vi "vol_path_by_id.get.vi"(8 "error in (no error)":errorcluster, 10 "vol id":i32, 11 "manager_daemon":refnum<class "manager_daemon.lvclass">) -> (0 "error out":errorcluster, 2 "Path":path, 3 "manager_daemon out":refnum<class "manager_daemon.lvclass">)   [LabVIEW 2024, in "manager_daemon.lvclass"]
uses:
  manager_daemon.lvclass
  manager_daemon.lvclass/manager_daemon.ctl
  type_defs/cmd--enum.ctl
  type_defs/msg--cluster.ctl
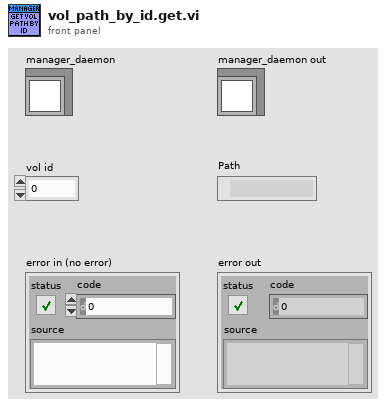
[diagram p1: front panel]
types:
  T1 = typedef "manager_daemon.lvclass/cmd--enum.ctl" = enum16{"init", "run", "load binaries", "build binaries", "save binaries", "return vol path by id", "display info", "apply filter", "add volume", "add issues", "add issue", "delete volume", "delete issues", "exit"}
  T2 = typedef "manager_daemon.lvclass/msg--cluster.ctl" = cluster{"cmd":T1, "data":variant}
  T3 = cluster{"vol id":i32, "notifier out":refnum<notifier>}
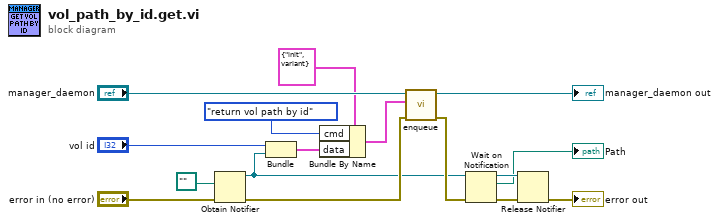
[diagram p0: block diagram]
diagram:
  n1 = Obtain Notifier(notification data type=path "", error in (no error)="error in (no error)") -> (notifier out=w5:refnum<notifier>, error out=w7:errorcluster)  [unwired: 2 in, 1 out]
  n2 = Bundle("vol id"="vol id", "notifier out"=w5) -> (w9:T3)  [unwired: 1 in]
  n3 = Bundle By Name(cluster=T2 {"cmd"=enum."init", "data"=variant} ("msg"), "cmd"=cmd--enum."return vol path by id", "data"=w9) -> (w11:T2)
  n4 = call "enqueue.vi"("error in (no error)"=w7, "msg"=w11, "manager_daemon in"="manager_daemon") -> ("error out"=w6:errorcluster, "manager_daemon out"=→"manager_daemon out":refnum<class "manager_daemon.lvclass">)  [unwired: 7 in]
  n5 = Wait on Notification(notifier=w5, error in (no error)=w6) -> (notifier out=w2:refnum<notifier>, notification=→"Path":path, error out=w4:errorcluster)  [unwired: 2 in, 1 out]
  n6 = Release Notifier(notifier=w2, error in (no error)=w4) -> (error out=→"error out":errorcluster)  [unwired: 1 in, 2 out]
